vi "Close Report File.vi"(8 "error in (no error)":errorcluster, 11 "Report In":refnum<class "Report Plugin.lvclass">) -> (0 "error out":errorcluster, 2 "Report Path":path)   [LabVIEW 2020, in "Report Plugin.lvclass"]
uses:
  Report Plugin.lvclass
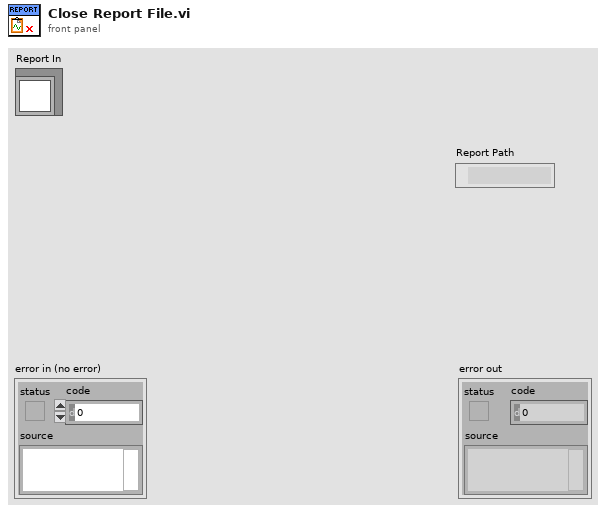
[diagram p1: front panel]
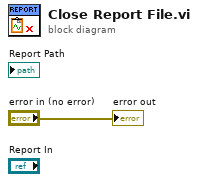
[diagram p0: block diagram]
diagram:
  "error out" <- "error in (no error)"
